vi "Nested Malleable VIs - Lesson 4.vi"() -> ()   [LabVIEW 2023]
doc: "Lesson 4 shows a way to protect your code when you have multiple malleable VIs that need almost the same parameterization, but where cross-wiring could result in code that is unbroken but logically incorrect."
uses:
  442a73b9-8abb-42ef-a319-57e943e9f4ee.vi
  a6bf1c3c-7dbe-4d9c-bdfa-97b8dc5b587e.vi
  ce2408b3-d287-497d-9e5c-238ab49fb6b8.vi
  442a73b9-8abb-42ef-a319-57e943e9f4ee.vi/5f008cf9-0835-42d5-ab12-715ade7a221f.vi
  a6bf1c3c-7dbe-4d9c-bdfa-97b8dc5b587e.vi/d4db2432-cc9c-482c-8957-dac855435ef6.vi
  a6bf1c3c-7dbe-4d9c-bdfa-97b8dc5b587e.vi/86fbf154-bd7b-49a2-8ab2-a837b2a95f24.vi
  a6bf1c3c-7dbe-4d9c-bdfa-97b8dc5b587e.vi/3b95b01e-1ec2-4565-bcd9-7606a5281010.vi
  a6bf1c3c-7dbe-4d9c-bdfa-97b8dc5b587e.vi/96a08935-737a-44b2-979c-a81d56408f7e.vi
  ce2408b3-d287-497d-9e5c-238ab49fb6b8.vi/5f008cf9-0835-42d5-ab12-715ade7a221f.vi
  442a73b9-8abb-42ef-a319-57e943e9f4ee.vi/5f008cf9-0835-42d5-ab12-715ade7a221f.vi/4a937600-749b-4ff4-8f55-34e6a7c3203b.vi
  a6bf1c3c-7dbe-4d9c-bdfa-97b8dc5b587e.vi/d4db2432-cc9c-482c-8957-dac855435ef6.vi/6eaecd13-6e48-4772-a921-b51ebdf84d88.vi
  a6bf1c3c-7dbe-4d9c-bdfa-97b8dc5b587e.vi/d4db2432-cc9c-482c-8957-dac855435ef6.vi/d2d5f2b7-06f4-47f6-971c-049c3fdbb653.vi
  a6bf1c3c-7dbe-4d9c-bdfa-97b8dc5b587e.vi/3b95b01e-1ec2-4565-bcd9-7606a5281010.vi/6eaecd13-6e48-4772-a921-b51ebdf84d88.vi
  a6bf1c3c-7dbe-4d9c-bdfa-97b8dc5b587e.vi/3b95b01e-1ec2-4565-bcd9-7606a5281010.vi/d2d5f2b7-06f4-47f6-971c-049c3fdbb653.vi
  a6bf1c3c-7dbe-4d9c-bdfa-97b8dc5b587e.vi/96a08935-737a-44b2-979c-a81d56408f7e.vi/6eaecd13-6e48-4772-a921-b51ebdf84d88.vi
  a6bf1c3c-7dbe-4d9c-bdfa-97b8dc5b587e.vi/96a08935-737a-44b2-979c-a81d56408f7e.vi/d2d5f2b7-06f4-47f6-971c-049c3fdbb653.vi
  ce2408b3-d287-497d-9e5c-238ab49fb6b8.vi/5f008cf9-0835-42d5-ab12-715ade7a221f.vi/4a937600-749b-4ff4-8f55-34e6a7c3203b.vi
panel:
  out "index of element 2\nINCORRECT":i32
  out "found 1":bool
  out "nearest index":i32
  out "index of element 1":i32
  # "Overview: This lesson shows a way to protect your code when you have multiple malleable VIs that need almost the same parameterization, but where cross-wiring could result in code that is unbroken but logically incorrect.\n\nInstructions: \n1. Open the block diagram of this VI. Review the lessons presented there.\n2. Run the VI to see the results. \n3. Once you have finished reviewing this VI, open the next lesson VI in the Malleable VIs - Nested Malleable VIs example project."
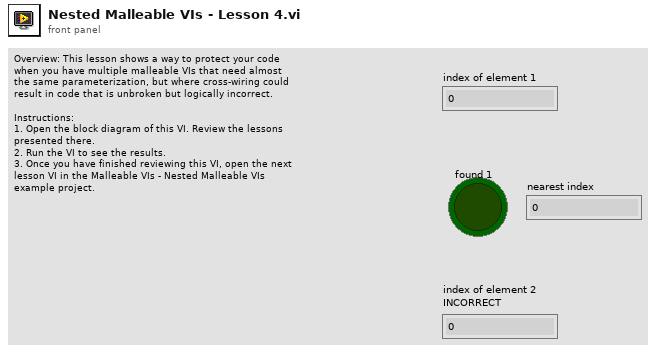
[diagram p1: front panel]
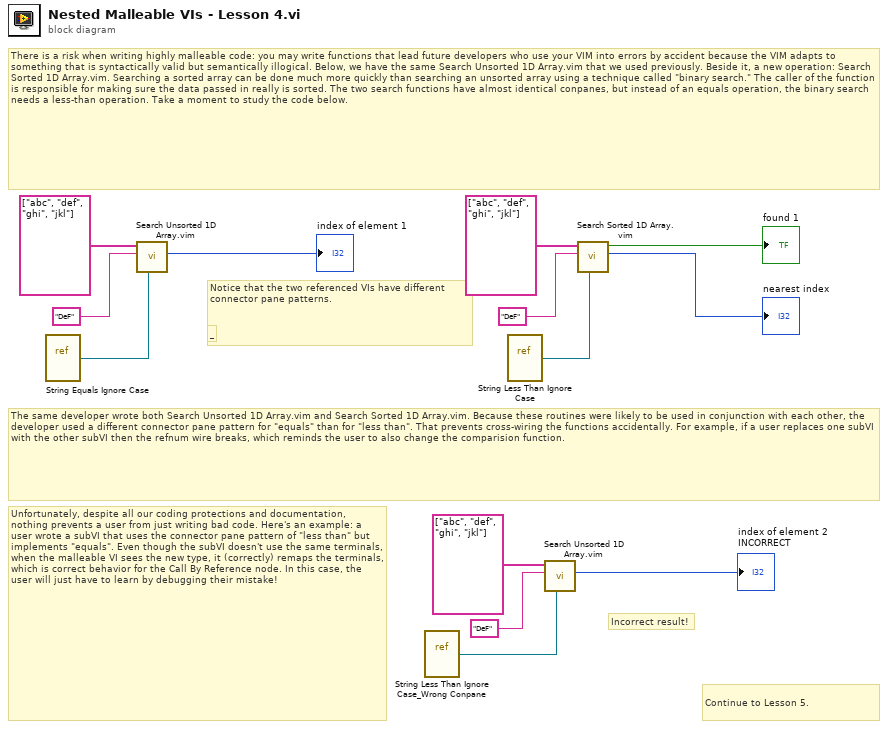
[diagram p0: block diagram]
diagram:
  # "Notice that the two referenced VIs have different connector pane patterns."
  # "Continue to Lesson 5."
  # "Incorrect result!"
  # "The same developer wrote both Search Unsorted 1D Array.vim and Search Sorted 1D Array.vim. Because these routines were likely to be used in conjunction with each other, the developer used a different connector pane pattern for \"equals\" than for \"less than\". That prevents cross-wiring the functions accidentally. For example, if a user replaces one subVI with the other subVI then the refnum wire breaks, which reminds the user to also change the comparision function."
  # "Unfortunately, despite all our coding protections and documentation, nothing prevents a user from just writing bad code. Here's an example: a user wrote a subVI that uses the connector pane pattern of \"less than\" but implements \"equals\". Even though the subVI doesn't use the same terminals, when the malleable VI sees the new type, it (correctly) remaps the terminals, which is correct behavior for the Call By Reference node. In this case, the user will just have to learn by debugging their mistake!"
  # "There is a risk when writing highly malleable code: you may write functions that lead future developers who use your VIM into errors by accident because the VIM adapts to something that is syntactically valid but semantically illogical. Below, we have the same Search Unsorted 1D Array.vim that we used previously. Beside it, a new operation: Search Sorted 1D Array.vim. Searching a sorted array can be done much more quickly than searching an unsorted array using a technique called \"binary search.\" The caller of the function is responsible for making sure the data passed in really is sorted. The two search functions have almost identical conpanes, but instead of an equals operation, the binary search needs a less-than operation. Take a moment to study the code below."
  # "_"
  n1 = vi-ref "String Equals Ignore Case.vi"() -> (w10:refnum<vi>)
  n2 = call "Search Unsorted 1D Array.vim"("equals function (built-in =)"=w10, "element"="DeF", "unsorted 1D array"=string[] ["abc", "def", "ghi", "jkl"] ("1D array")) -> ("index of element"=→"index of element 1":i32)  [unwired: 8 in]
  n3 = vi-ref "String Less Than Ignore Case_Wrong Conpane.vi"() -> (w4:refnum<vi>)
  n4 = vi-ref "String Less Than Ignore Case.vi"() -> (w5:refnum<vi>)
  n5 = call "Search Unsorted 1D Array.vim"("equals function (built-in =)"=w4, "element"="DeF", "unsorted 1D array"=string[] ["abc", "def", "ghi", "jkl"] ("1D array")) -> ("index of element"=→"index of element 2\nINCORRECT":i32)  [unwired: 8 in]
  n6 = call "Search Sorted 1D Array.vim"("less function (built-in <)"=w5, "element"="DeF", "sorted 1D array"=string[] ["abc", "def", "ghi", "jkl"] ("1D array")) -> ("nearest index"=→"nearest index":i32, "found?"=→"found 1":bool)  [unwired: 7 in]
